vi "Plot Format 3D Surface.vi"(6 "Units":string, 8 "Data 2D Table":cluster{"X":sgl[], "Y":sgl[], "Z":sgl[][]}, 11 "3D Surface":refnum<vi>) -> ()   [LabVIEW 2016]
uses:
  <vilib>/Math Plots/3D Math Plots/3D Surface/3D Surface XCtrl/3D Surface.xctl
  <vilib>/Math Plots/3D Math Plots/3D Surface/3D Surface Datatype/Public/Plot Helper (Vector).vi
  <vilib>/Math Plots/3D Math Plots/3D Surface/3D Surface Datatype/3D Surface Datatype.lvclass
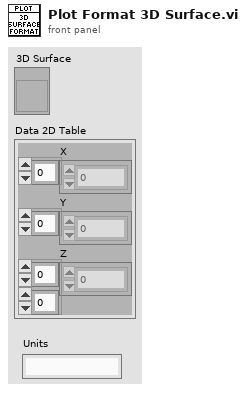
[diagram p1: front panel]
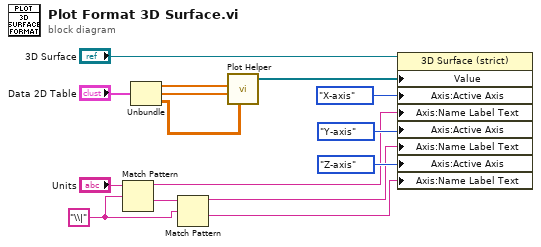
[diagram p0: block diagram]
diagram:
  w4 = "\\|" ("regular expression")
  n1 = Match Pattern(string="Units", regular expression=w4) -> (before substring=w3:string, after substring=w6:string)  [unwired: 1 in, 2 out]
  n2 = Unbundle("Data 2D Table") -> ("X"=w12:sgl[], "Y"=w11:sgl[], "Z"=w10:sgl[][])
  n3 = Match Pattern(string=w6, regular expression=w4) -> (before substring=w2:string, after substring=w1:string)  [unwired: 1 in, 2 out]
  n4 = call-poly <vilib>:"Plot Helper.vi"("z matrix"=w10, "y vector"=w11, "x vector"=w12) -> ("3D Plot lvclass Array out"=w14:refnum<class "3D Plot Datatype.lvclass">[])  [unwired: 3 in, 5 out]
  n5 = property class="3D Surface (strict)"(reference="3D Surface", "Value"=w14, "Axis:Active Axis"=enum16{"X-axis", "Y-axis", "Z-axis"}."X-axis", "Axis:Name Label Text"=w3, "Axis:Active Axis"=enum16{"X-axis", "Y-axis", "Z-axis"}."Y-axis", "Axis:Name Label Text"=w2, "Axis:Active Axis"=enum16{"X-axis", "Y-axis", "Z-axis"}."Z-axis", "Axis:Name Label Text"=w1) -> ()  [unwired: 1 in, 2 out]
